vi "get_number_of_pulses.vi"(8 "error in (no error)":errorcluster, 11 "GenericClock.lvclass in":refnum<class "GenericClock.lvclass">) -> (0 "error out":errorcluster, 2 "number of pulses":i32, 3 "GenericClock.lvclass out":refnum<class "GenericClock.lvclass">)   [LabVIEW 2010, in "GenericClock.lvclass"]
uses:
  GenericClock/GenericClock/GenericClock.lvclass
  GenericClock/GenericClock/GenericClock.lvclass/GenericClock.ctl
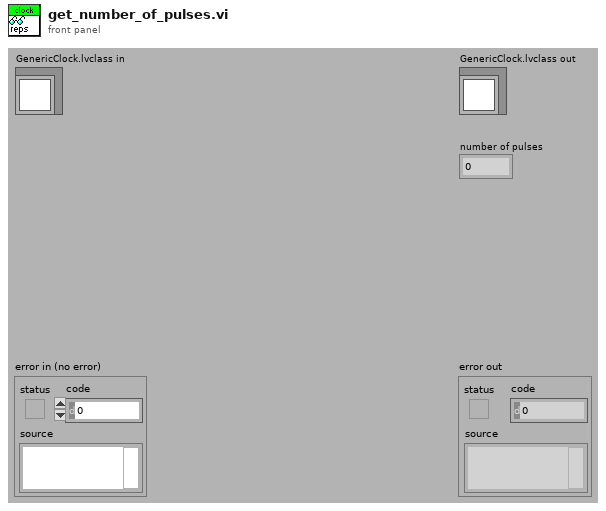
[diagram p1: front panel]
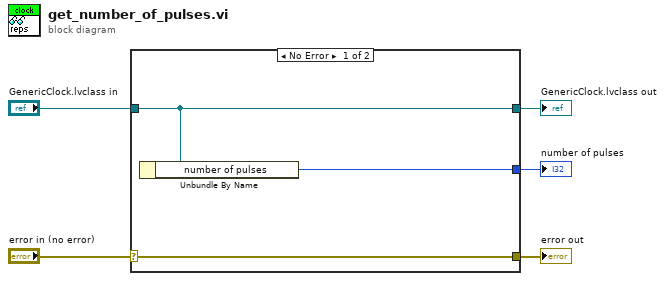
[diagram p0: block diagram]
diagram:
  n1 = case shown="No Error" "error in (no error)" {
    selector: "error in (no error)" -> [w8 w9]
    tunnel: [w8 w9] -> w4
    tunnel: [w7 w10] -> w2
    tunnel: "GenericClock.lvclass in" -> [w7 w10]
    tunnel: [w6 _] -> w1
    frame No Error {
      n2 = Unbundle By Name(w7) -> ("number of pulses"=w6:u32)
    }
    frame Error {
    }
  }
  "error out" <- w4
  "GenericClock.lvclass out" <- w2
  "number of pulses" <- w1
